vi "runtime path validation.vi"(8 "error in":errorcluster, 11 "TDMS datalogger configuration in":refnum<class "TDMS datalogger configuration.lvclass">) -> (0 "error out":errorcluster, 3 "TDMS datalogger configuration out":refnum<class "TDMS datalogger configuration.lvclass">)   [LabVIEW 2015, in "TDMS datalogger configuration.lvclass"]
uses:
  TDMS datalogger configuration.lvclass
  TDMS datalogger configuration.lvclass/TDMS datalogger configuration.ctl
  Write log directory.vi
  Write log name.vi
  Read backup directory.vi
  Write backup directory.vi
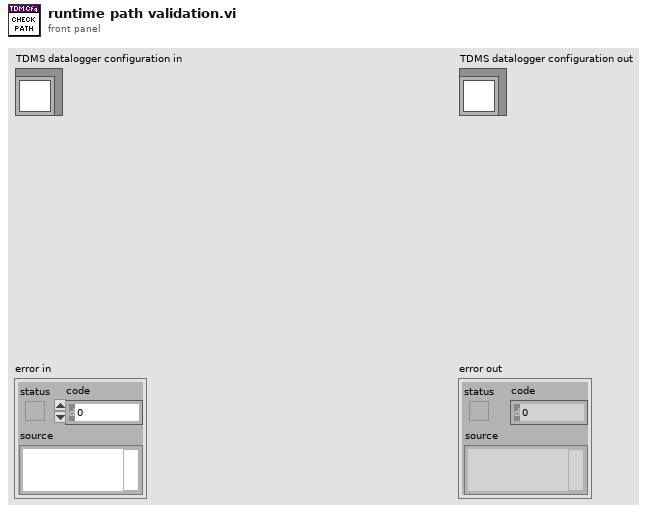
[diagram p1: front panel]
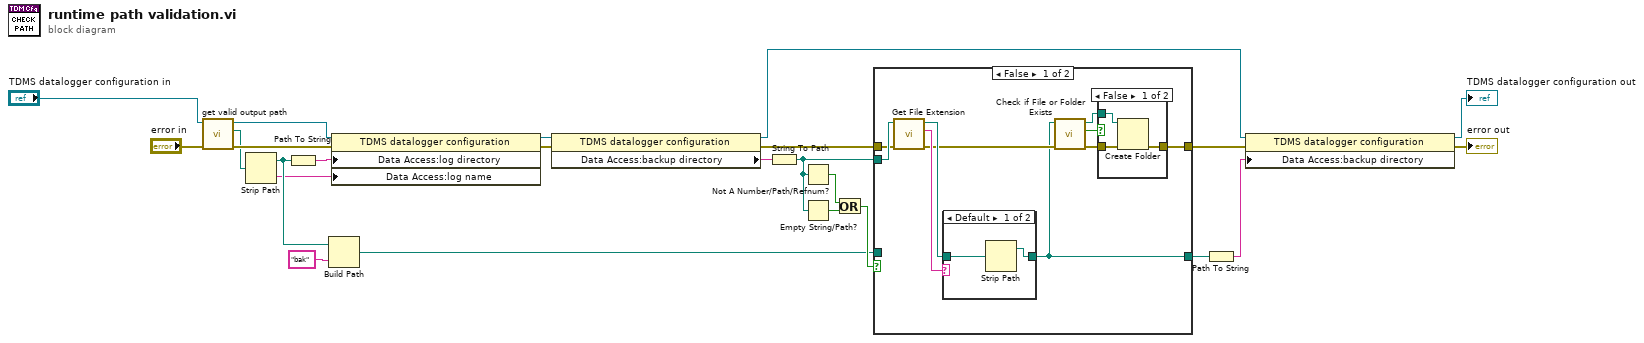
[diagram p0: block diagram]
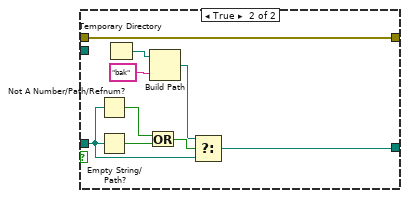
[diagram p4: hidden frame]
diagram:
  n1 = call "get valid output path.vi"("error in (no error)"="error in", "TDMS datalogger configuration in"="TDMS datalogger configuration in") -> ("error out"=w20:errorcluster, "Path"=w8:path, "TDMS datalogger configuration out"=w19:refnum<class "TDMS datalogger configuration.lvclass">)  [unwired: 7 in]
  n2 = Strip Path(path=w8) -> (stripped path=w4:path, name=w3:string)
  n3 = Path To String(path=w4) -> (string=w5:string)
  n4 = Build Path(base path=w4, name or relative path="bak") -> (appended path=w6:path)
  n5 = property class="TDMS datalogger configuration"(reference=w19, error in=w20, "Data Access:log directory"=w5, "Data Access:log name"=w3) -> (reference out=w22:refnum<class "TDMS datalogger configuration.lvclass">, error out=w21:errorcluster)
  n6 = property class="TDMS datalogger configuration"(reference=w22, error in=w21) -> (reference out=w10:refnum<class "TDMS datalogger configuration.lvclass">, error out=w14:errorcluster, "Data Access:backup directory"=w15:string)
  n7 = String To Path(string=w15) -> (path=w2:path)
  n8 = Not A Number/Path/Refnum?(number/path/refnum=w2) -> (NaN/Path/Refnum?=w17:bool)
  n9 = Empty String/Path?(string/path=w2) -> (empty?=w18:bool)
  n10 = Or(x=w17, y=w18) -> (x .or. y?=w16:bool)
  n11 = case shown="False" w16 {
    tunnel: [w25 w44] -> w12
    tunnel: [w30 w49] -> w13
    tunnel: w2 -> [w27 _]
    tunnel: w14 -> [w26 w49]
    tunnel: w6 -> [_ w43]
    frame False {
      n12 = call <vilib>:"Get File Extension.vi"("error in (no error)"=w26, "file"=w27) -> ("error out"=w32:errorcluster, "lowercase file extension"=w33:string, "dup file"=w34:path)  [unwired: 5 in, 2 out]
      n13 = case shown="Default" w33 {
        tunnel: w34 -> [w40 w41]
        tunnel: [w39 w41] -> w25
        frame Default {
          n14 = Strip Path(path=w40) -> (stripped path=w39:path)  [unwired: 1 out]
        }
        frame "" {
        }
      }
      n15 = call <vilib>:"Check if File or Folder Exists.vi"("error in (no error)"=w32, "path"=w25) -> ("error out"=w29:errorcluster, "file or folder exists?"=w31:bool, "dup path"=w28:path)  [unwired: 7 in]
      n16 = case shown="False" w31 {
        tunnel: [w35 w38] -> w30
        tunnel: w29 -> [w36 w38]
        tunnel: w28 -> [w37 _]
        frame False {
          n17 = Create Folder(path (use dialog)=w37, error in=w36) -> (error out=w35:errorcluster)  [unwired: 1 in, 2 out]
        }
        frame True {
        }
      }
    }
    frame True {
      n18 = Not A Number/Path/Refnum?(number/path/refnum=w43) -> (NaN/Path/Refnum?=w48:bool)
      n19 = Empty String/Path?(string/path=w43) -> (empty?=w47:bool)
      n20 = Temporary Directory() -> (w50:path)
      n21 = Or(x=w48, y=w47) -> (x .or. y?=w46:bool)
      n22 = Build Path(base path=w50, name or relative path="bak") -> (appended path=w45:path)
      n23 = Select(t=w45, s=w46, f=w43) -> (s? t:f=w44:path)
    }
  }
  n24 = Path To String(path=w12) -> (string=w1:string)
  n25 = property class="TDMS datalogger configuration"(reference=w10, error in=w13, "Data Access:backup directory"=w1) -> (reference out=→"TDMS datalogger configuration out":refnum<class "TDMS datalogger configuration.lvclass">, error out=→"error out":errorcluster)
